vi "Insight Write Message.vi"(1 "User Data":string, 2 "Position":u8, 3 "Line":enum16{"LINE_1", "LINE_2"}(ring), 4 "I2CDevRef":T1 {"Device Address" format="%.0x"}) -> ()   [LabVIEW 2012]
uses:
  <vilib>/Rock Robotics/WPI/I2C/WPI_I2CDevRef.ctl
  <vilib>/Rock Robotics/SystemInterfaces/Typedef/FPGA_TypedefDigitalModule.ctl
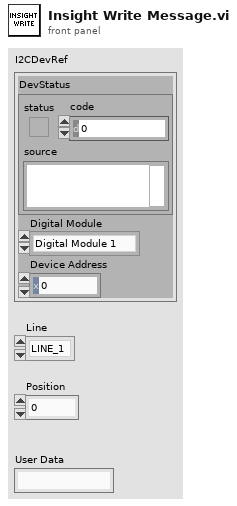
[diagram p1: front panel]
types:
  T1 = typedef "WPI_I2CDevRef.ctl" = cluster{"DevStatus":errorcluster, "Digital Module":T2, "Device Address":u8}
  T2 = typedef "FPGA_TypedefDigitalModule.ctl" = enum16{"Digital Module 1", "Digital Module 2"}
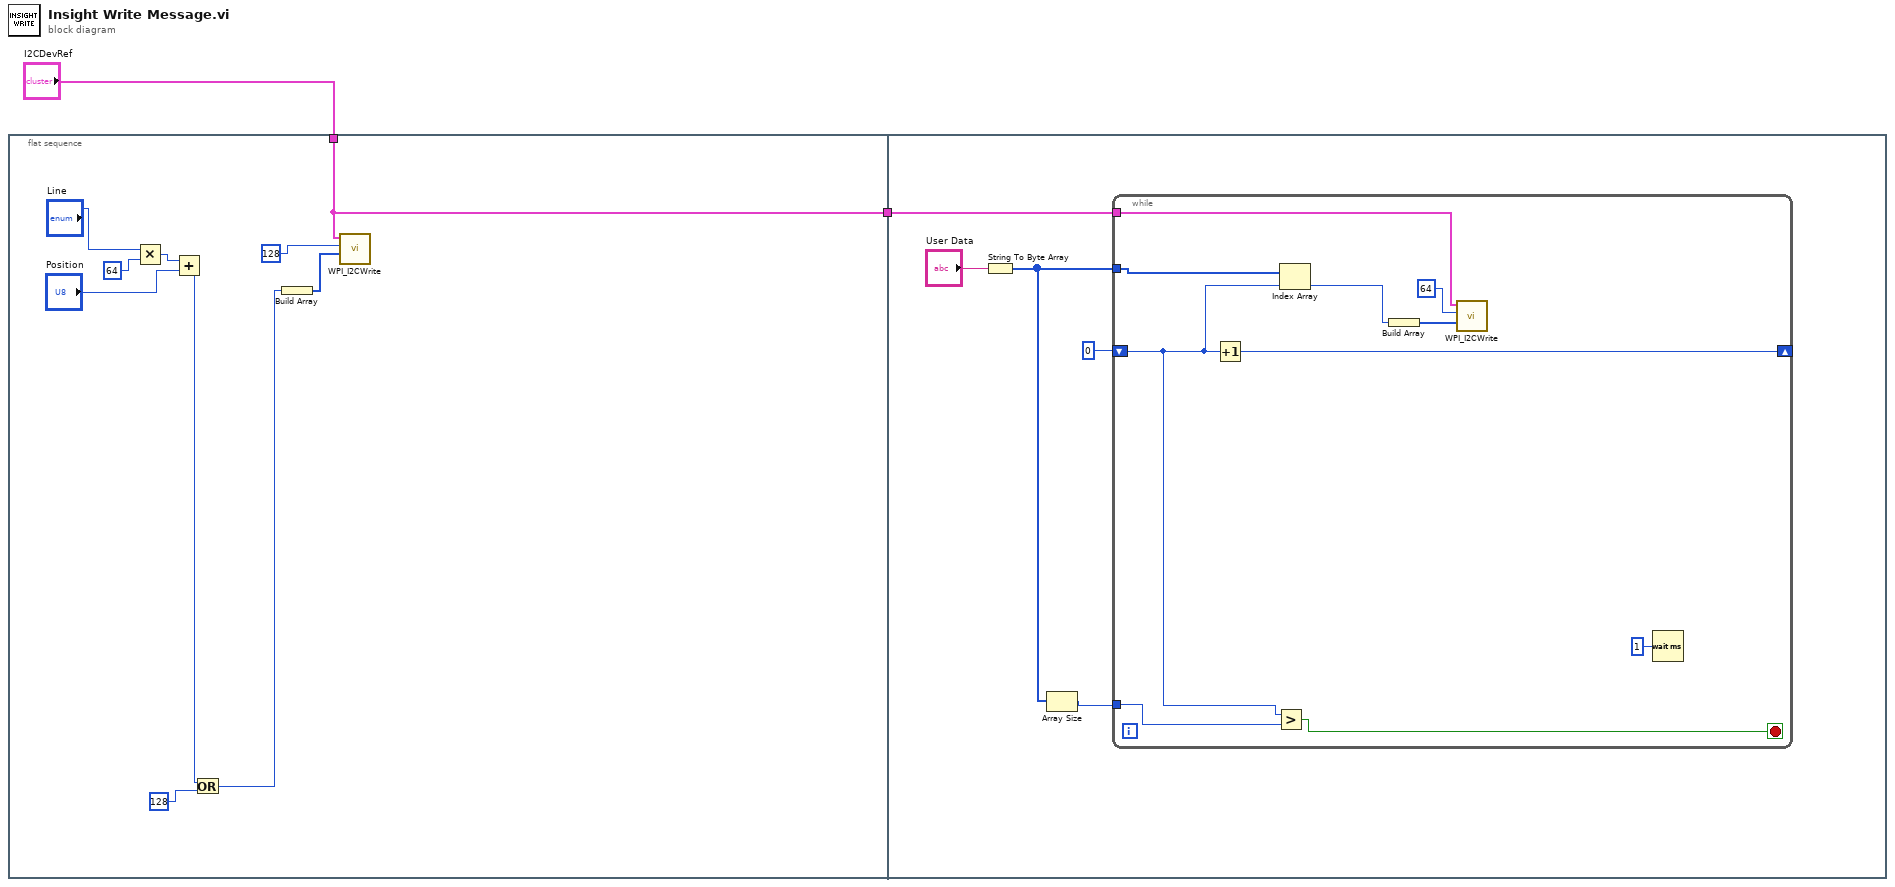
[diagram p0: block diagram]
diagram:
  n1 = flat-sequence {
    tunnel: "I2CDevRef" -> [w3]
    tunnel: [w3] -> w1
    tunnel: w1 -> [w13]
    frame #0 {
      n2 = Multiply(x="Line", y=u8 64 ("element")) -> (x*y=w9:u16)
      n3 = Add(x=w9, y="Position") -> (x+y=w11:u16)
      n4 = Or(x=w11, y=u8 128 ("element")) -> (x .or. y?=w6:u16)
      n5 = Build Array(w6) -> (w5:u16[])
      n6 = call <vilib>:"WPI_I2CWrite.vi"("I2CDataToSend"=w5, "I2CRegister"=u8 128 ("element"), "I2CDevRef"=w3) -> ()  [unwired: 7 in, 2 out]
    }
    frame #1 {
      n7 = String To Byte Array(string="User Data") -> (unsigned byte array=w14:u8[])
      n8 = Array Size(array=w14) -> (size(s)=w15:i32)
      n9 = while {
        shift-right: [w26] -> _
        shift-left: 0 ("Numeric") -> [w21]
        tunnel: w15 -> [w27]
        tunnel: w14 -> [w25]
        tunnel: w13 -> [w19]
        stop <- w20 stop-if-true
        n10 = Increment(x=w21) -> (x+1=w26:i32)
        n11 = Greater?(x=w21, y=w27) -> (0:w20:bool)
        n12 = Index Array(array=w25, index=w21) -> (element=w22:u8)
        n13 = Build Array(w22) -> (w23:u8[])
        n14 = call <vilib>:"WPI_I2CWrite.vi"("I2CDataToSend"=w23, "I2CRegister"=u8 64 ("element"), "I2CDevRef"=w19) -> ()  [unwired: 7 in, 2 out]
        n15 = Wait (ms)(milliseconds to wait=u32 1) -> ()  [unwired: 1 out]
      }
    }
  }
